vi "Target Choice to position x,y.vi"(10 "Array":T1(array[cluster]), 11 "Target Choice":i8(knob) scale=0.0..2.0) -> (1 "Distance [m]":dbl, 2 "Numeric Target Info (X,Y,D)":dbl[](array[numeric]), 3 "Position of Target Center X":dbl, 4 "Center Target":bool, 5 "Position of Target Center Y":dbl)   [LabVIEW 2012]
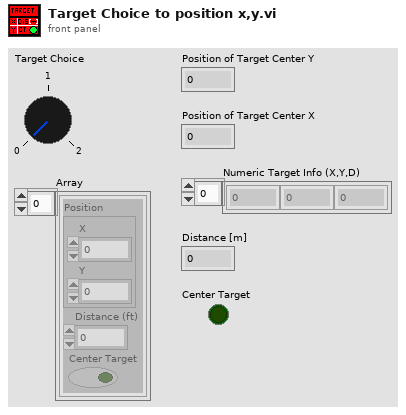
[diagram p1: front panel]
types:
  T1 = cluster{"Position":cluster{"X":dbl, "Y":dbl}, "Distance (ft)":dbl, "Center Target":bool}[]
  T2 = cluster{"Position":cluster{"X":dbl, "Y":dbl}, "Distance (ft)":dbl, "Center Target":bool}
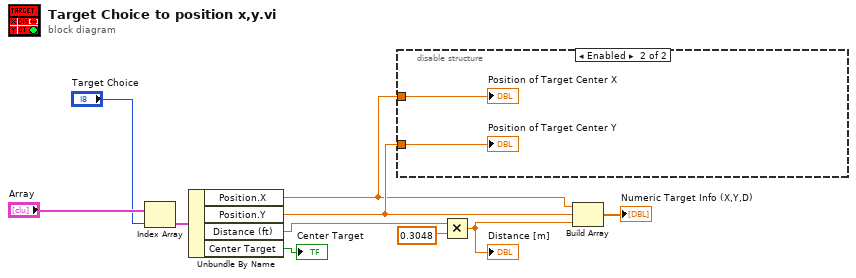
[diagram p0: block diagram]
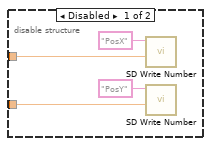
[diagram p2: hidden frame]
diagram:
  n1 = Index Array(array="Array", index="Target Choice") -> (element=w9:T2)
  n2 = Unbundle By Name(w9) -> ("Position.X"=w6:dbl, "Position.Y"=w7:dbl, "Distance (ft)"=w5:dbl, "Center Target"=→"Center Target":bool)
  n3 = disable-structure shown="Enabled" {
    disable-tunnel: w6 -> [w12 w16]
    disable-tunnel: w7 -> [w11 w15]
    frame Disabled {
      n4 = call <vilib>:"SD Write Number.vi"("Numeric"=w12, "Name"="PosX") -> ()  [unwired: 8 in, 2 out]
      n5 = call <vilib>:"SD Write Number.vi"("Numeric"=w11, "Name"="PosY") -> ()  [unwired: 8 in, 2 out]
    }
    frame Enabled {
      "Position of Target Center X" <- w16
      "Position of Target Center Y" <- w15
    }
  }
  n6 = Multiply(x=w5, y=0.3048) -> (x*y=w8:dbl)
  "Distance [m]" <- w8
  n7 = Build Array(w6, w7, w8) -> (→"Numeric Target Info (X,Y,D)":dbl[])
